vi "P2-5.vi"() -> ()   [LabVIEW 2011]
panel:
  out "숫자형 2":dbl
  in  "숫자형":dbl
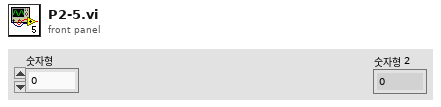
[diagram p1: front panel]
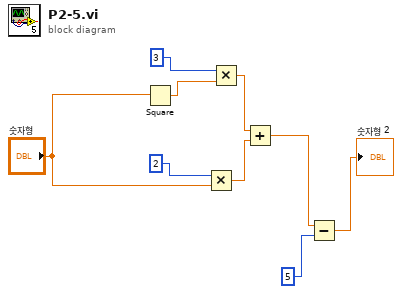
[diagram p0: block diagram]
diagram:
  n1 = Square(x="숫자형") -> (x^2=w8:dbl)
  n2 = Multiply(x=2, y="숫자형") -> (x*y=w5:dbl)
  n3 = Multiply(x=3, y=w8) -> (x*y=w4:dbl)
  n4 = Add(x=w4, y=w5) -> (x+y=w3:dbl)
  n5 = Subtract(x=w3, y=5) -> (x-y=→"숫자형 2":dbl)
